vi "Set_Rev_history_params_mass.vi"() -> ()   [LabVIEW 2014]
panel:
  out "Processed Vis":string
  in  "path 2":path
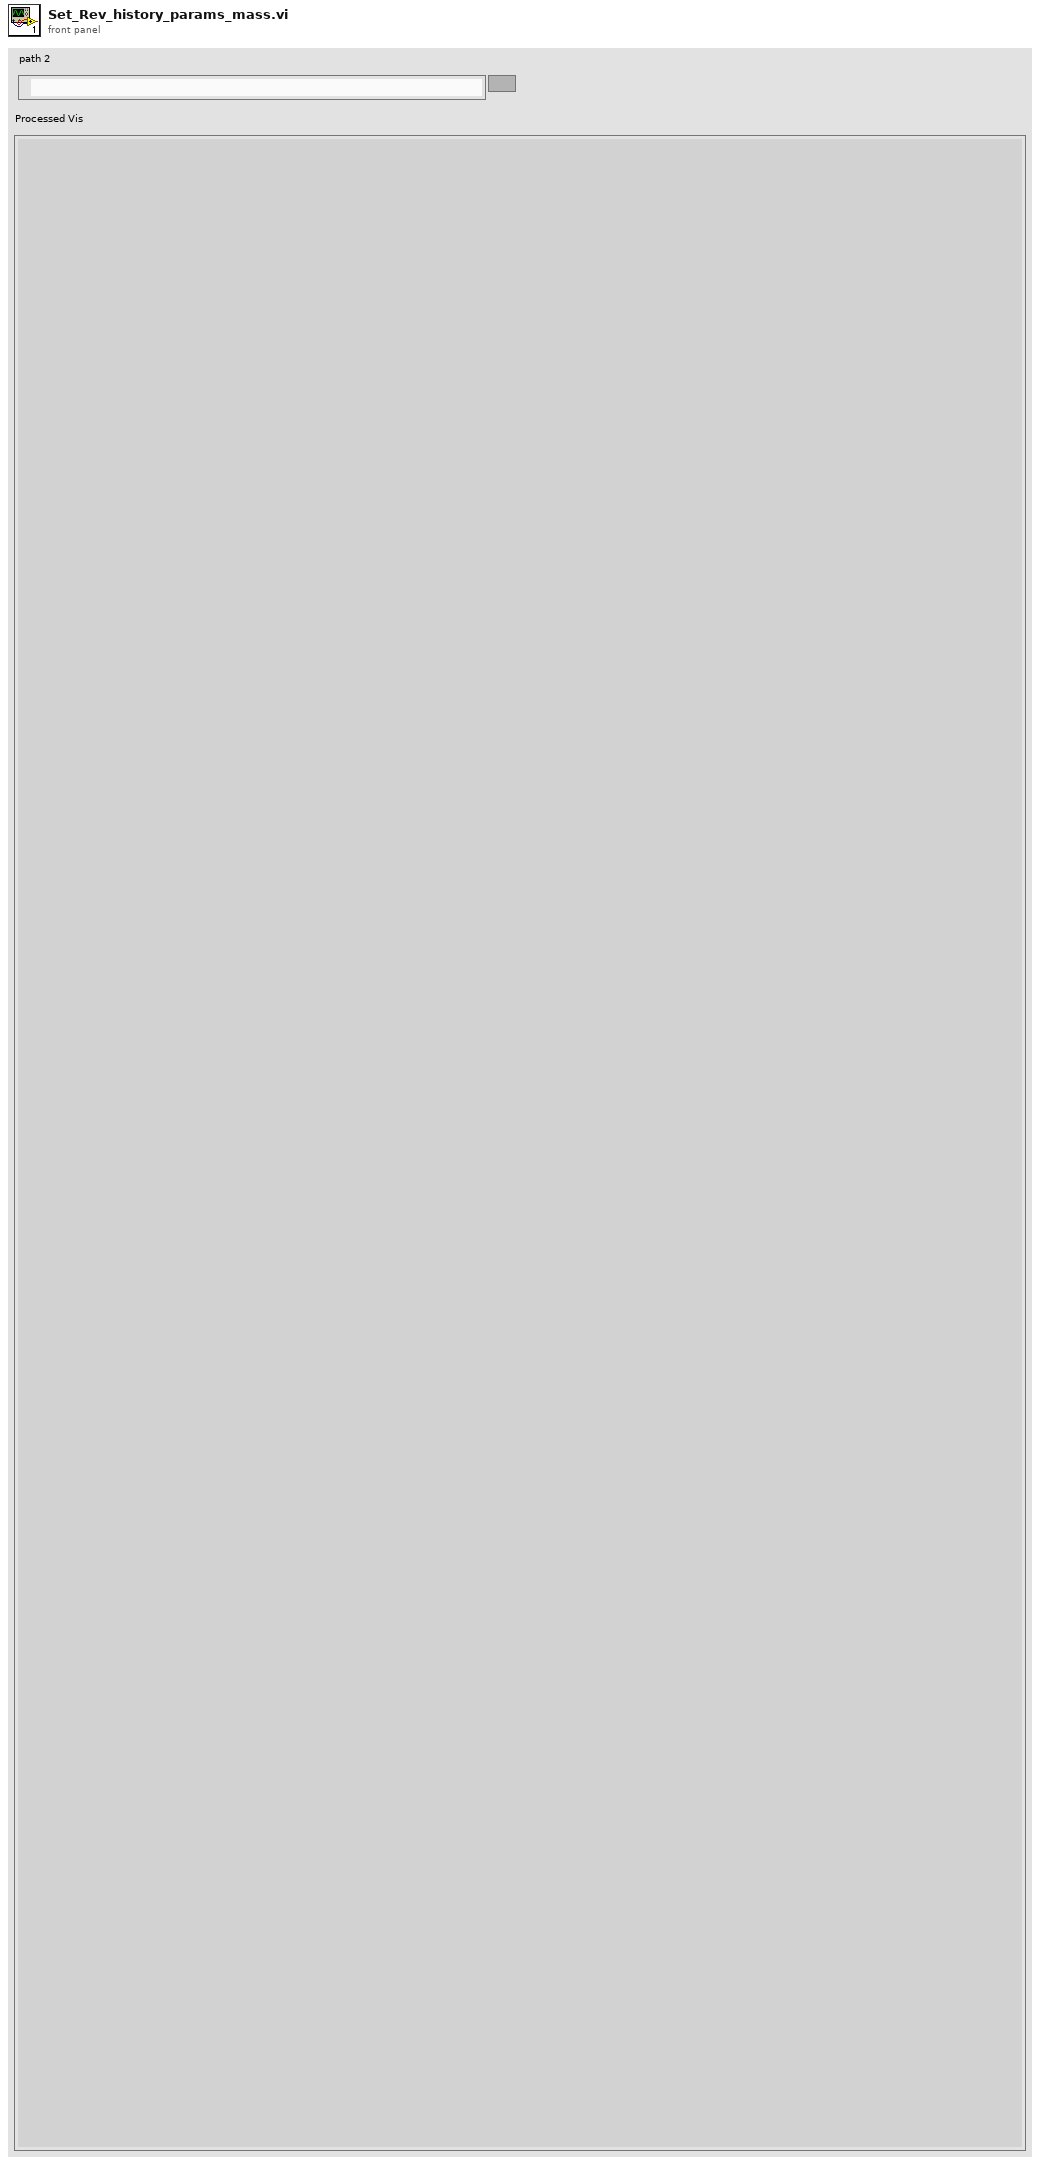
[diagram p1: front panel]
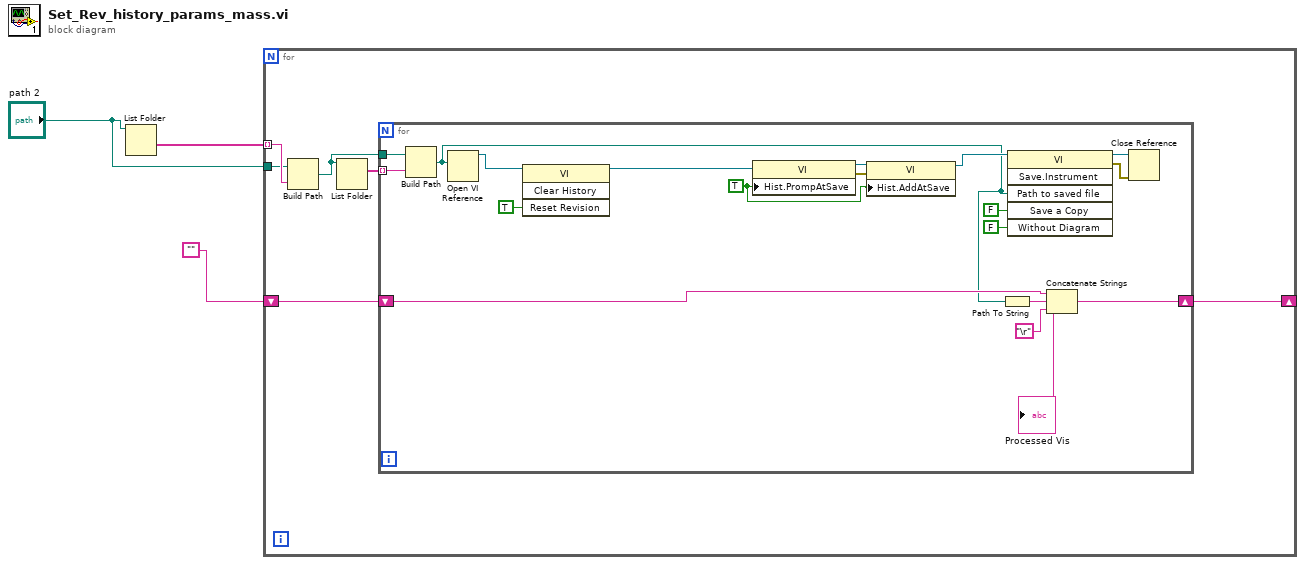
[diagram p0: block diagram]
diagram:
  n1 = List Folder(path="path 2") -> (folder names=w3:string[])  [unwired: 3 in, 3 out]
  n2 = for {
    tunnel: w3 -> [w7] mode=indexing
    tunnel: "path 2" -> [w6]
    shift-right: [w4] -> _
    shift-left: "" -> [w5]
    n3 = Build Path(base path=w6, name or relative path=w7) -> (appended path=w8:path)
    n4 = List Folder(path=w8) -> (filenames=w9:string[])  [unwired: 3 in, 3 out]
    n5 = for {
      tunnel: w9 -> [w27] mode=indexing
      tunnel: w8 -> [w26]
      shift-right: [w10] -> w4
      shift-left: w5 -> [w14]
      w18 = TRUE ("History:Prompt for Comments At Save")
      n6 = Build Path(base path=w26, name or relative path=w27) -> (appended path=w13:path)
      n7 = Open VI Reference(vi path=w13) -> (vi reference=w24:refnum<vi>)  [unwired: 5 in, 1 out]
      n8 = invoke class="VI" method="Clear History"(reference=w24, "Reset Revision"=TRUE) -> (reference out=w21:refnum<vi>)  [unwired: 2 in, 3 out]
      n9 = property class="VI"(reference=w21, "Hist.PrompAtSave"=w18) -> (reference out=w20:refnum<vi>, error out=w19:errorcluster)  [unwired: 1 in]
      n10 = property class="VI"(reference=w20, error in=w19, "Hist.AddAtSave"=w18) -> (reference out=w17:refnum<vi>)  [unwired: 1 out]
      n11 = Path To String(path=w13) -> (string=w12:string)
      n12 = invoke class="VI" method="Save.Instrument"(reference=w17, "Path to saved file"=w13, "Save a Copy"=FALSE, "Without Diagram"=FALSE) -> (reference out=w15:refnum<vi>, error out=w16:errorcluster)  [unwired: 2 in, 4 out]
      n13 = Concatenate Strings(w14, w12, "\r") -> (w10:string)
      "Processed Vis" <- w10
      n14 = Close Reference(reference=w15, error in (no error)=w16) -> ()  [unwired: 1 out]
    }
  }
